vi "Read Array Key (String).vi"(6 "Read Raw String? (F)":bool, 7 "Section Name":string, 8 "error in (no error)":errorcluster, 10 "Key Name":string, 11 "Config in":refnum<class "LabVIEW-Config.lvclass">) -> (0 "error out":errorcluster, 1 "Value":string[](array[string]), 2 "Key Found?":bool, 3 "Config out":refnum<class "LabVIEW-Config.lvclass">)   [LabVIEW 2017, in "LabVIEW-Config.lvlib" / "LabVIEW-Config.lvclass"]
uses:
  LabVIEW-Config.lvclass
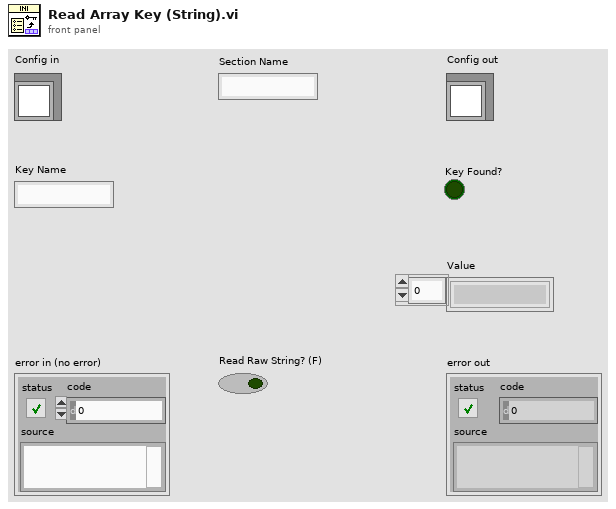
[diagram p1: front panel]
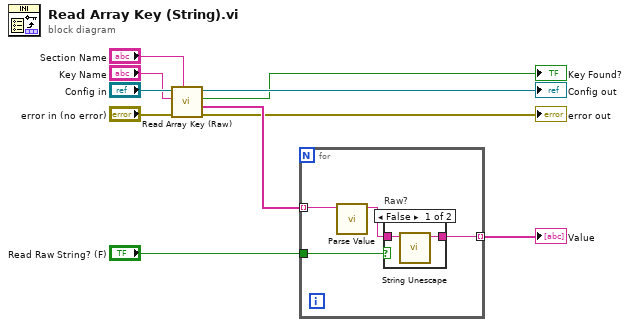
[diagram p0: block diagram]
diagram:
  n1 = call "Read Array Key (Raw).vi"("Section Name"="Section Name", "error in (no error)"="error in (no error)", "Key Name"="Key Name", "Config in"="Config in") -> ("error out"=→"error out":errorcluster, "Content"=w5:string[], "Key Found?"=→"Key Found?":bool, "Config out"=→"Config out":refnum<class "LabVIEW-Config.lvclass">)  [unwired: 4 in]
  n2 = for {
    tunnel: w5 -> [w14] mode=indexing
    tunnel: [w13] -> w3 mode=indexing
    tunnel: "Read Raw String? (F)" -> [w12]
    n3 = call "Parse Value.vi"("Value"=w14) -> ("Value (Quotes Removed)"=w11:string)  [unwired: 9 in, 1 out]
    n4 = case "Raw?" shown="False" w12 {
      tunnel: w11 -> [w16 w17]
      tunnel: [w15 w17] -> w13
      frame False {
        n5 = call "String Unescape.vi"("Escaped String"=w16) -> ("Unescaped String"=w15:string)  [unwired: 10 in]
      }
      frame True {
      }
    }
  }
  "Value" <- w3
